vi "T_FlipFlop.vi"(2 "CLK":bool, 3 "T":bool) -> (0 "__\nQ":bool, 1 "Q":bool)   [LabVIEW 2018]
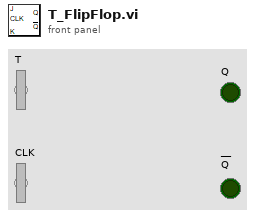
[diagram p1: front panel]
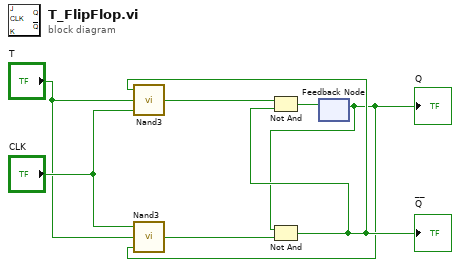
[diagram p0: block diagram]
diagram:
  n1 = feedback #1() -> (w2:bool)  [unwired: 1 in]
  "Q" <- w2
  n2 = call "Nand3.vi"("C"=w2, "B"="T", "A"="CLK") -> ("Boolean"=w6:bool)
  n3 = Not And(1:w6, 2:w2) -> (0:w3:bool)
  "__\nQ" <- w3
  n4 = call "Nand3.vi"("C"="CLK", "B"="T", "A"=w3) -> ("Boolean"=w5:bool)
  n5 = Not And(1:w3, 2:w5) -> (0:w7:bool)
  n6 = feedback-in #1(w7) -> ()
